vi "Send DI Data Queue.vi"(4 "error in":errorcluster, 6 "DI Waveforms":bool[][](array[boolean])) -> (0 "error out":errorcluster)   [LabVIEW 2020]
uses:
  DAQ Engine VIs/PXI Globals.vi
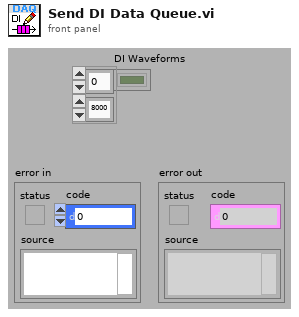
[diagram p1: front panel]
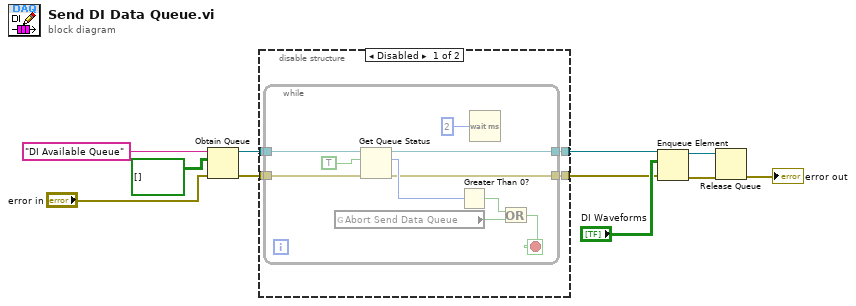
[diagram p0: block diagram]
diagram:
  n1 = Obtain Queue(name (unnamed)="DI Available Queue", element data type=bool[][] [] ("AI Waveforms 2"), error in (no error)="error in") -> (queue out=w4:refnum<queue>, error out=w2:errorcluster)  [unwired: 2 in, 1 out]
  n2 = disable-structure shown="Disabled" {
    disable-tunnel: w4 -> [w15 w27]
    disable-tunnel: [w14 w27] -> w3
    disable-tunnel: w2 -> [w13 w26]
    disable-tunnel: [w12 w26] -> w1
    frame Disabled {
      n3 = while {
        tunnel: w15 -> [w19]
        tunnel: [w18] -> w14
        tunnel: w13 -> [w17]
        tunnel: [w16] -> w12
        stop <- w22 stop-if-true
        n4 = global read "PXI Globals.vi" "Abort Send Data Queue"() -> (w20:bool)
        n5 = Get Queue Status(queue=w19, return elements? (F)=TRUE, error in (no error)=w17) -> (queue out=w18:refnum<queue>, # pending remove=w23:i32, error out=w16:errorcluster)  [unwired: 5 out]
        n6 = Greater Than 0?(x=w23) -> (x > 0?=w21:bool)
        n7 = Wait (ms)(milliseconds to wait=2) -> ()  [unwired: 1 out]
        n8 = Or(x=w21, y=w20) -> (x .or. y?=w22:bool)
      }
    }
    frame Enabled {
    }
  }
  n9 = Enqueue Element(queue=w3, element="DI Waveforms", error in (no error)=w1) -> (queue out=w6:refnum<queue>, error out=w5:errorcluster)  [unwired: 1 in, 1 out]
  n10 = Release Queue(queue=w6, error in (no error)=w5) -> (error out=→"error out":errorcluster)  [unwired: 1 in, 2 out]
